vi "PH_Cont-601k_PSU.PC Config.vi"(0 "VI in":refnum<vi>, 2 "Configuration":T1 items=["Ch intl, Fl intl, QSw intl", "Ch intl, Fl intl, QSw ext", "Ch intl, Fl ext, QSw intl", "Ch intl, Fl ext, QSw ext", "Ch ext, Fl int, QSw int", "Ch ext, Fl int, QSw ext", "Ch ext, Fl ext, QSw int", "Ch ext, Fl ext, QSw ext"], 5 "error in (no error)":errorcluster) -> (14 "VI out":refnum<vi>, 17 "\"Config\" changed":bool, 19 "error out":errorcluster)   [LabVIEW 2014, in "PH_Cont-601k_PSU.lvlib"]
uses:
  PH_Cont-601k_PSU.lvlib
  PH_Cont-601k_PSU.Configuration.ctl
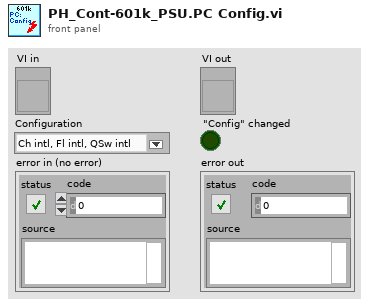
[diagram p1: front panel]
types:
  T1 = typedef "PH_Cont-601k_PSU.lvlib/PH_Cont-601k_PSU.Configuration.ctl" = u16
  T2 = typedef "PH_Cont-601k_PSU.lvlib/PH_Cont-601k_PSU.i attribute.ctl" = cluster{"GUI Refs":T3, "Interlock":bool, "Service ID applied Voltage":i32, "Device Settings":cluster{"Configuration":T1, "Flash Interval [s]":dbl, "Mode":T4, "Voltage [V]":u16, "Charge":bool, "VISA resource name":refnum<visa-resource-name>}, "Readyness":T5, "Information":cluster{"VISA resource name":refnum<visa-resource-name>, "Tagname Power On":string, "Interlock":cluster{"Instance":string, "Tagname":string}, "Limits [V]":cluster{"Lower":dbl, "Upper":dbl}, "Tagname PSU On":string}, "R2S":bool, "Charge is allowed":bool}
  T3 = typedef "PH_Cont-601k_PSU.lvlib/PH_Cont-601k_PSU.GUI Refs.ctl" = cluster{"Power On":refnum<vi>, "Hard- and Software":refnum<vi>, "Device Status":refnum<vi>, "Device Error":refnum<vi>, "Configuration":refnum<vi>, "Flash Interval [s]":refnum<vi>, "Interlock":refnum<vi>, "Interlock Indicator":refnum<vi>, "Voltage [V]":refnum<vi>, "Readyness":refnum<vi>, "Mode":refnum<vi>, "Reset Error":refnum<vi>, "Expert working":refnum<vi>, "Charge":refnum<vi>, "PSU On":refnum<vi>}
  T4 = typedef "PH_Cont-601k_PSU.lvlib/PH_Cont-601k_PSU.Mode.ctl" = enum32{"STOP", "STANDBY", "READY", "EMISSION", "ERROR"}
  T5 = typedef "PH_Cont-601k_PSU.lvlib/PH_Cont-601k_PSU.Readyness.ctl" = cluster{"Program":T6, "Device":T7}
  T6 = typedef "PH_Cont-601k_PSU.lvlib/PH_Cont-601k_PSU.Readyness Program.ctl" = enum32{"OFF", "POWER", "INTERLOCK"}
  T7 = typedef "PH_Cont-601k_PSU.lvlib/PH_Cont-601k_PSU.Readyness Device.ctl" = enum32{"OFF", "CONNECTING", "CONNECTED", "OPERATING", "EOC", "ERROR"}
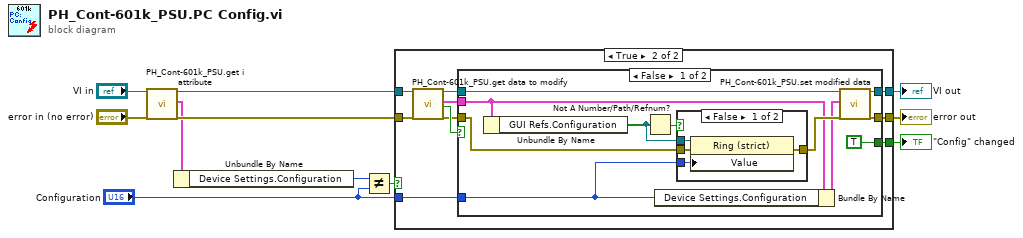
[diagram p0: block diagram]
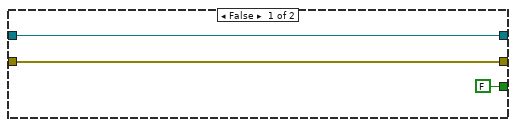
[diagram p2: hidden frame]
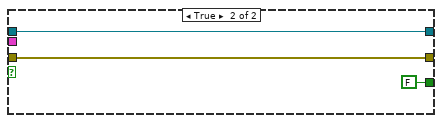
[diagram p4: hidden frame]
diagram:
  n1 = call "PH_Cont-601k_PSU.get i attribute.vi"("i ref in"="VI in", "error in (no error)"="error in (no error)") -> ("i ref out"=w6:refnum<vi>, "i attribute"=w5:T2, "error out"=w8:errorcluster)  [unwired: 15 in]
  n2 = Unbundle By Name(w5) -> ("Device Settings.Configuration"=w4:T1)
  n3 = Not Equal?(x=w4, y="Configuration") -> (x != y?=w3:bool)
  n4 = case shown="True" w3 {
    tunnel: [w13 w24] -> w11
    tunnel: [w14 w23] -> w10
    tunnel: w8 -> [w13 w18]
    tunnel: w6 -> [w14 w17]
    tunnel: "Configuration" -> [_ w16]
    tunnel: [FALSE w15] -> w1
    frame False {
    }
    frame True {
      n5 = call "PH_Cont-601k_PSU.get data to modify.vi"("i ref in"=w17, "error in (no error)"=w18) -> ("i ref out"=w20:refnum<vi>, "i attribute"=w21:T2, "timed out"=w22:bool, "error out"=w19:errorcluster)  [unwired: 14 in]
      n6 = case shown="False" w22 {
        tunnel: [w30 w42] -> w24
        tunnel: w19 -> [w29 w42]
        tunnel: w20 -> [w35 w43]
        tunnel: [w31 w43] -> w23
        tunnel: w21 -> [w33 _]
        tunnel: w16 -> [w28 _]
        tunnel: [TRUE FALSE] -> w15
        frame False {
          n7 = Unbundle By Name(w33) -> ("GUI Refs.Configuration"=w26:refnum<vi>)
          n8 = Not A Number/Path/Refnum?(number/path/refnum=w26) -> (NaN/Path/Refnum?=w27:bool)
          n9 = Bundle By Name(cluster=w33, "Device Settings.Configuration"=w28) -> (w32:T2)
          n10 = case shown="False" w27 {
            tunnel: [w39 w40] -> w34
            tunnel: w26 -> [w38 _]
            tunnel: w29 -> [w37 w40]
            tunnel: w28 -> [w36 _]
            frame False {
              n11 = property class="Ring (strict)"(reference=w38, error in=w37, "Value"=w36) -> (error out=w39:errorcluster)  [unwired: 1 out]
            }
            frame True {
            }
          }
          n12 = call "PH_Cont-601k_PSU.set modified data.vi"("i ref in"=w35, "i attribute"=w32, "error in (no error)"=w34) -> ("i ref out"=w31:refnum<vi>, "error out"=w30:errorcluster)  [unwired: 15 in]
        }
        frame True {
        }
      }
    }
  }
  "error out" <- w11
  "VI out" <- w10
  "\"Config\" changed" <- w1
